vi "to_json.vi"(8 "error in":errorcluster, 11 "dataset in":refnum<class "dataset.lvclass">) -> (0 "error out":errorcluster, 2 "json":string, 3 "dataset out":refnum<class "dataset.lvclass">, 4 "Not Default":bool)   [LabVIEW 2020, in "datasources.lvlib" / "dataset.lvclass"]
uses:
  dataset.lvclass
  dataset.lvclass/dataset.ctl
  706ce30a-5b81-48c0-969a-66c87b7b4567.vi
  d062dd61-71d6-44b5-8ec0-c8fc7e52ec0a.vi
  datasetName.get.vi
  datasetDescription.get.vi
  <vilib>/JDP Science/JSONtext/Variant to JSON Text.vi
  <vilib>/JDP Science/JSONtext/LVClass Serializer/JSONtext LVClass Serializer.lvclass
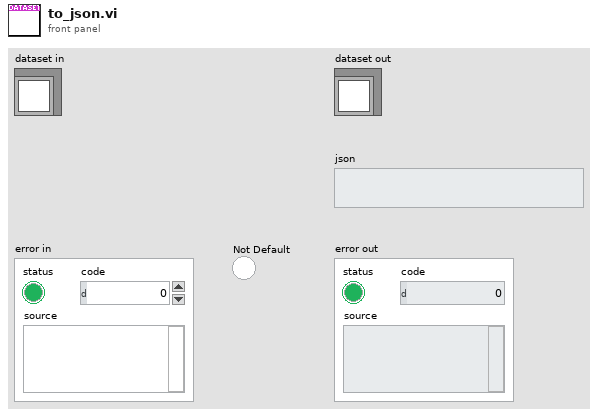
[diagram p1: front panel]
types:
  T1 = cluster{"datasetName":string, "datasetDescription":string}
  T2 = cluster{"datasetName":bool, "datasetDescription":bool}
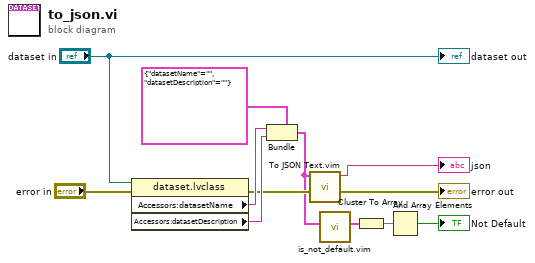
[diagram p0: block diagram]
diagram:
  n1 = property class="dataset.lvclass"(reference="dataset in", error in="error in") -> (error out=w6:errorcluster, "Accessors:datasetName"=w11:string, "Accessors:datasetDescription"=w10:string)  [unwired: 1 out]
  n2 = Bundle(cluster=T1 {"datasetName"="", "datasetDescription"=""}, "datasetName"=w11, "datasetDescription"=w10) -> (w4:T1)
  n3 = call "To JSON Text.vim"("error in (no error)"=w6, "Anything"=w4) -> ("error out"=→"error out":errorcluster, "<JSON>"=→"json":string)  [unwired: 8 in]
  n4 = call "is_not_default.vim"("data"=w4) -> ("Not Default"=w3:T2)  [unwired: 10 in]
  n5 = Cluster To Array(cluster=w3) -> (array=w2:bool[])
  n6 = And Array Elements(Boolean array=w2) -> (logical AND=→"Not Default":bool)
  "dataset out" <- "dataset in"
